vi "InitTable.vi"(8 "Error In":errorcluster, 11 "Table 2":refnum<vi>) -> (0 "Error Out":errorcluster)   [LabVIEW 2014]
uses:
  Controls/ColumnHeaders1.ctl
panel:
  in  "ColumnHeaders":T1
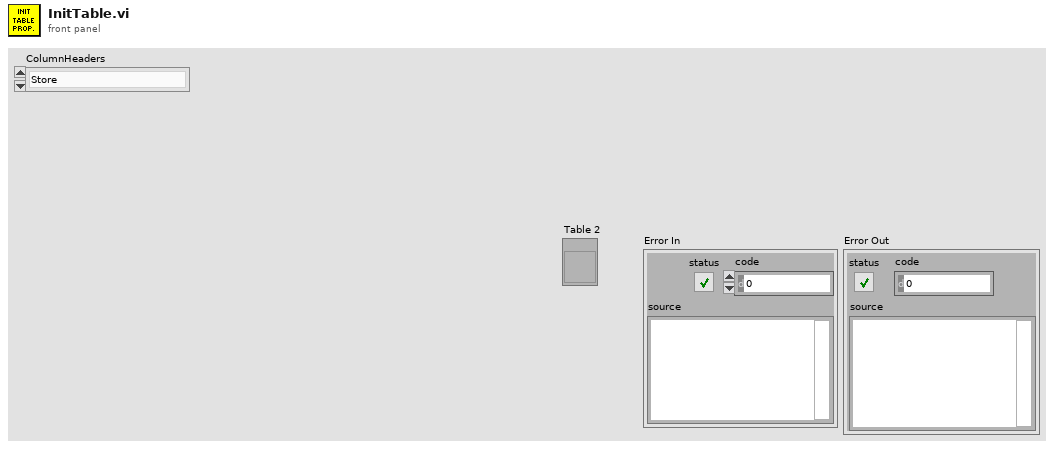
[diagram p1: front panel]
types:
  T1 = typedef "ColumnHeaders1.ctl" = enum16{"Store", "Display", "Method", "Property", "Unit", "URL", "IP Address", "Data Block", "Address", "Data Type"}
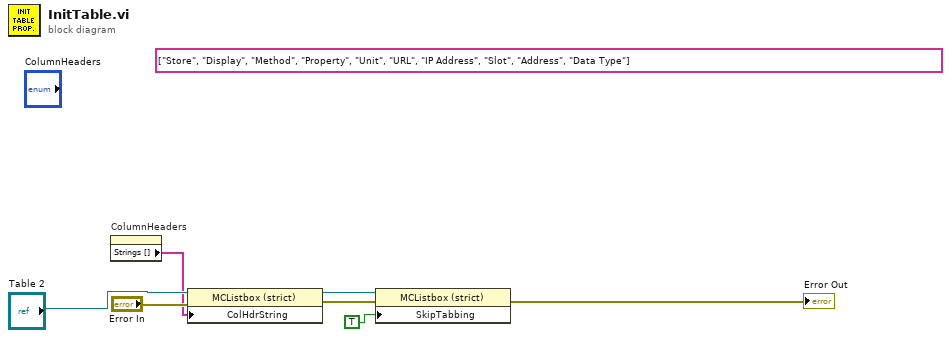
[diagram p0: block diagram]
diagram:
  (unwired) string[] ["Store", "Display", "Method", "Property", "Unit", "URL", "IP Address", "Slot", "Address", "Data Type"] ("Column Header Strings[]")
  n1 = property on="ColumnHeaders" class="Enum (strict)"() -> ("Strings []"=w1:string[])  [unwired: 2 in, 2 out]
  n2 = property on="Property Node" class="MCListbox (strict)"(reference="Table 2", error in="Error In", "ColHdrString"=w1) -> (reference out=w7:refnum<vi>, error out=w6:errorcluster)
  n3 = property on="Property Node" class="MCListbox (strict)"(reference=w7, error in=w6, "SkipTabbing"=TRUE ("Skip When Tabbing")) -> (error out=→"Error Out":errorcluster)  [unwired: 1 out]
